vi "Instrument Manager Loop.vi"(8 "System Control":refnum<queue>, 11 "Instrument Manager":refnum<queue>) -> (0 "error out":errorcluster)   [LabVIEW 2020, in "ChromTech Series I Pump.lvlib" / "Instrument Manager.lvlib"]
uses:
  Instrument Manager/Instrument Manager.lvlib
  support/Message Queue/Message Cluster.ctl
  Instrument Manager/Instrument State.ctl
  <vilib>/Utility/error.llb/Error Cluster From Error Code.vi
  <vilib>/ErrorRing/Error Ring.xnode
  support/Message Queue/Message Queue.lvlib
  ChromTech Series I Pump.lvlib
  <instrlib>/RxnRover/ChromtechSeriesIDriver/ChromTech Series I Drivers.lvlib
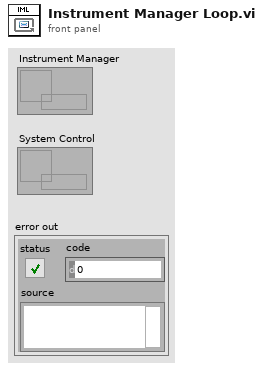
[diagram p1: front panel]
types:
  T1 = typedef "ChromTech Series I Pump.lvlib/Instrument Manager.lvlib/Instrument State.ctl" = cluster{"VISA Resource":refnum<visa-resource-name>, "Flow Rate":dbl, "Running":bool, "Running Since":timestamp, "Pressure Data Point":cluster{"Time Stamp":timestamp, "Value":dbl}, "Upper Pressure Fault":bool, "Lower Pressure Fault":bool, "Motor Stall Fault":bool, "Sampling Rate (sec/sample)":dbl, "Retry Attempts":i32, "Fast Comms":bool}
  T2 = cluster{"seconds since 1Jan1904":timestamp, "Pressure":dbl}
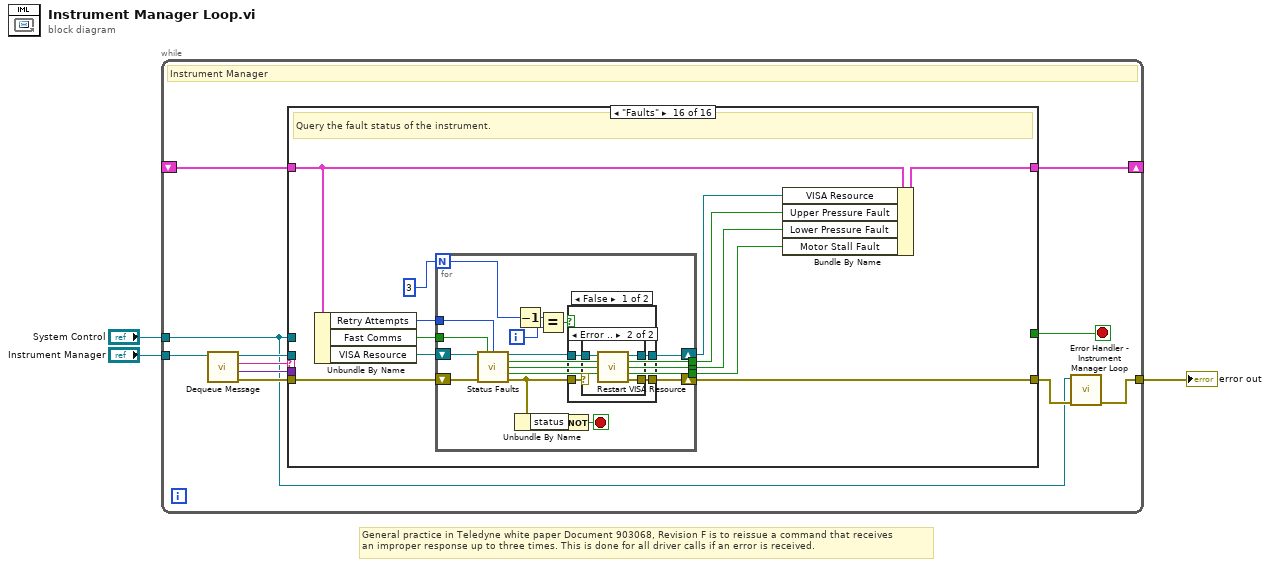
[diagram p0: block diagram]
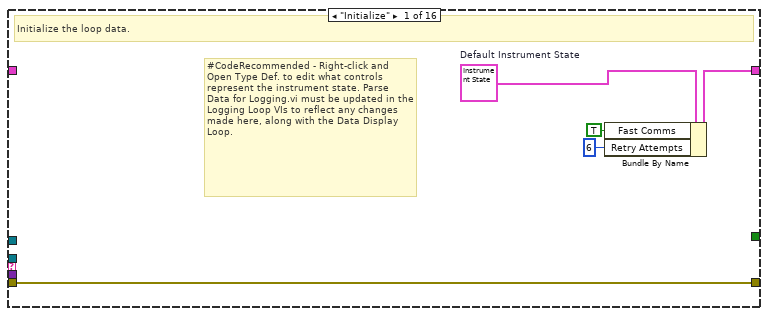
[diagram p2: hidden frame]
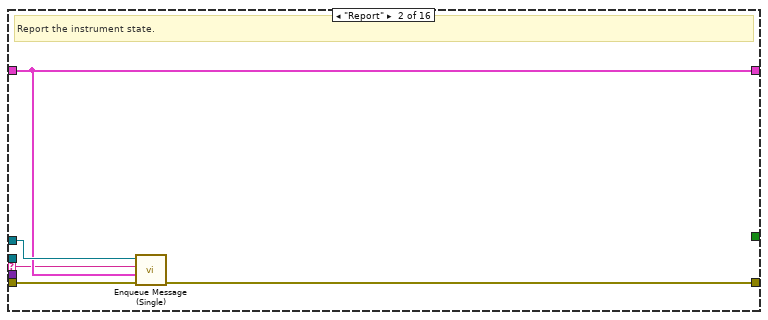
[diagram p3: hidden frame]
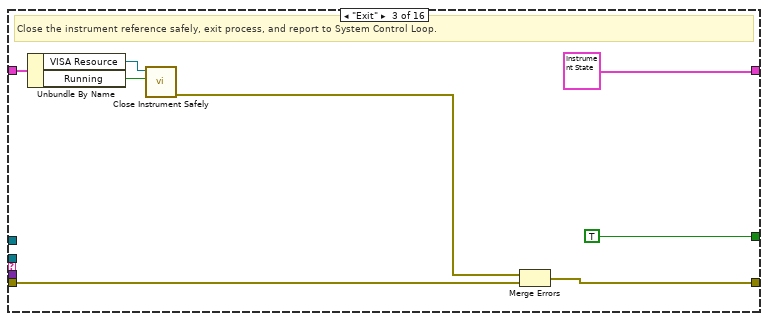
[diagram p4: hidden frame]
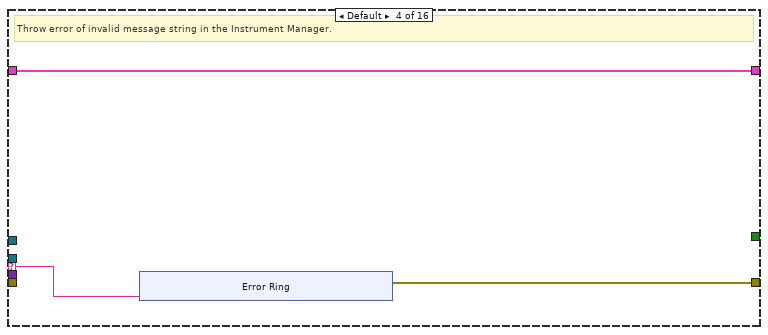
[diagram p5: hidden frame]
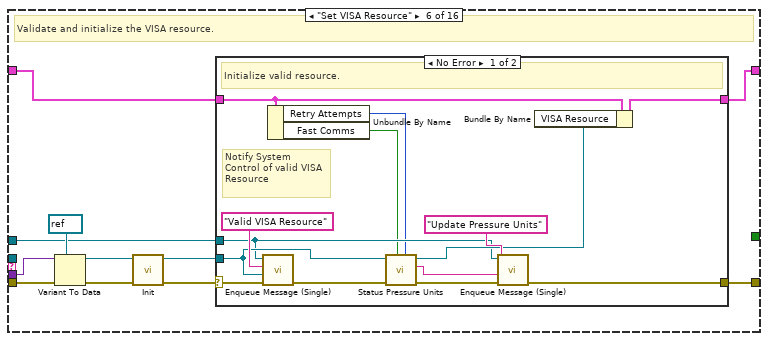
[diagram p7: hidden frame]
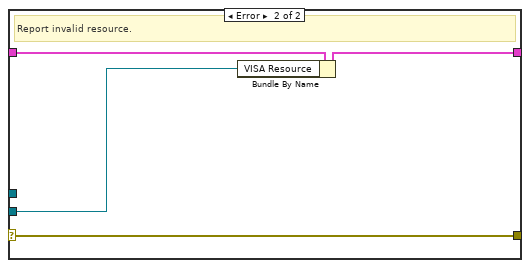
[diagram p8: hidden frame]
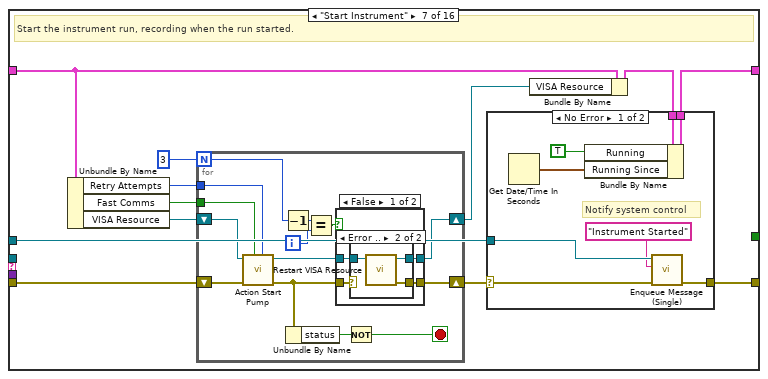
[diagram p9: hidden frame]
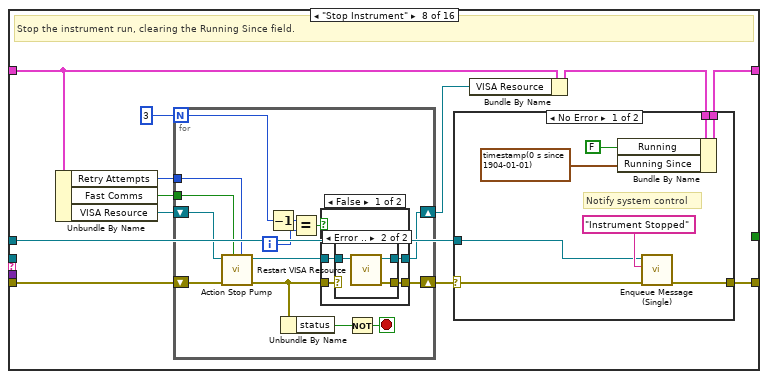
[diagram p13: hidden frame]
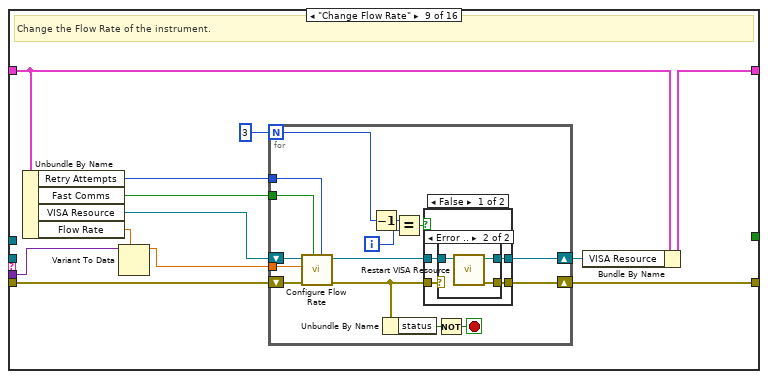
[diagram p17: hidden frame]
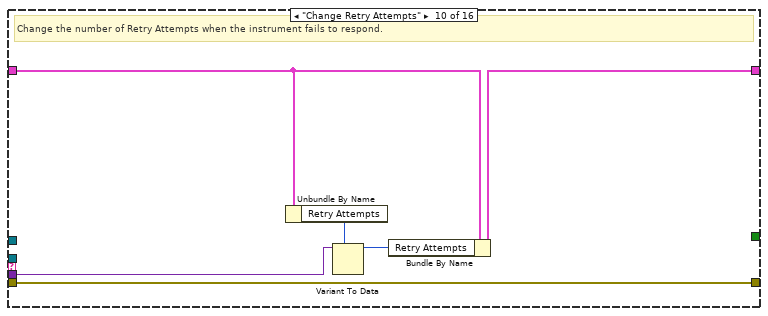
[diagram p20: hidden frame]
diagram:
  # "General practice in Teledyne white paper Document 903068, Revision F is to reissue a command that receives\nan improper response up to three times. This is done for all driver calls if an error is received."
  n1 = while {
    tunnel: "Instrument Manager" -> [w14]
    tunnel: "System Control" -> [w4]
    tunnel: [w8] -> w1
    shift-right: [w6] -> _
    shift-left: _ -> [w7]
    stop <- w5 stop-if-true
    # "Instrument Manager"
    n2 = call "Dequeue Message.vi"("Message Queue"=w14) -> ("error out"=w10:errorcluster, "Message Data"=w11:variant, "Message"=w13:string, "dup Message Queue"=w12:refnum<queue>)  [unwired: 7 in]
    n3 = case shown="\"Faults\"" w13 {
      selector: w13 -> [_ w20 _ w34 _ _ _ _ _ _ _ _ _ _ _ _]
      tunnel: w12 -> [_ _ _ _ _ _ _ _ _ _ _ _ _ _ _ _]
      tunnel: w4 -> [_ w23 _ _ _ w45 w84 w131 _ _ _ _ _ _ _ _]
      tunnel: w11 -> [_ _ _ _ _ w52 _ _ w178 w210 w216 _ _ _ _ _]
      tunnel: w10 -> [w18 w24 w27 _ w43 w51 w82 w129 w173 w207 w213 w220 w229 w264 w304 w342]
      tunnel: [w18 w22 w26 w33 w43 w55 w85 w132 w172 w207 w213 w220 w228 w263 w302 w340] -> w9
      tunnel: w7 -> [_ w21 w32 w35 w44 w54 w81 w127 w177 w209 w215 w219 w227 w265 w301 w339]
      tunnel: [w17 w21 T1 {"VISA Resource"="", "Flow Rate"=0.0, "Running"=FALSE, "Running Since"=timestamp(0 s since 1904-01-01), "Pressure Data Point"={"Time Stamp"=timestamp(0 s since 1904-01-01), "Value"=0.0}, "Upper Pressure Fault"=FALSE, "Lower Pressure Fault"=FALSE, "Motor Stall Fault"=FALSE, "Sampling Rate (sec/sample)"=0.0, "Retry Attempts"=0, "Fast Comms"=FALSE} w35 w44 w53 w83 w130 w179 w211 w217 w219 w230 w268 w303 w341] -> w6
      tunnel: [_ _ TRUE _ _ _ _ _ _ _ _ _ _ _ _ _] -> w5
      frame "Initialize" {
        w19 = T1 {"VISA Resource"="", "Flow Rate"=0.0, "Running"=FALSE, "Running Since"=timestamp(0 s since 1904-01-01), "Pressure Data Point"={"Time Stamp"=timestamp(0 s since 1904-01-01), "Value"=0.0}, "Upper Pressure Fault"=FALSE, "Lower Pressure Fault"=FALSE, "Motor Stall Fault"=FALSE, "Sampling Rate (sec/sample)"=0.0, "Retry Attempts"=0, "Fast Comms"=FALSE}  # Default Instrument State
        # "#CodeRecommended - Right-click and Open Type Def. to edit what controls represent the instrument state. Parse Data for Logging.vi must be updated in the Logging Loop VIs to reflect any changes made here, along with the Data Display Loop."
        # "Initialize the loop data."
        n4 = Bundle By Name(cluster=w19, "Fast Comms"=TRUE, "Retry Attempts"=6) -> (w17:T1)
      }
      frame "Report" {
        # "Report the instrument state."
        n5 = call "Enqueue Message (Single).vi"("error in (no error)"=w24, "Message Data"=w21, "Message"=w20, "Message Queue"=w23) -> ("error out"=w22:errorcluster)  [unwired: 6 in, 1 out]
      }
      frame "Exit" {
        # "Close the instrument reference safely, exit process, and report to System Control Loop."
        n6 = Unbundle By Name(w32) -> ("VISA Resource"=w30:refnum<visa-resource-name>, "Running"=w31:bool)
        n7 = call "Close Instrument Safely.vi"("Running (F)"=w31, "VISA Refnum in"=w30) -> ("error out"=w25:errorcluster)  [unwired: 9 in]
        n8 = Merge Errors(w25, w27) -> (w26:errorcluster)
      }
      frame Default {
        # "Throw error of invalid message string in the Instrument Manager."
        n9 = xnode "Error Ring"("parameter 0"=w34) -> ("error out"=w33:errorcluster)
      }
      frame "--- Copy This Frame ---" {
        # "Copy this frame and add responses to instrument specific messages."
      }
      frame "Set VISA Resource" {
        # "Validate and initialize the VISA resource."
        n10 = Variant To Data(error in=w51, type=refnum<visa-resource-name> refnum, Variant=w52) -> (data=w49:refnum<visa-resource-name>, error out=w50:errorcluster)
        n11 = call "Init.vi"("error in (no error)"=w50, "VISA resource in"=w49) -> ("error out"=w46:errorcluster, "VISA resource out"=w47:refnum<visa-resource-name>)  [unwired: 8 in]
        n12 = case shown="No Error" w46 {
          selector: w46 -> [w69 w70]
          tunnel: w47 -> [w62 w71]
          tunnel: [w64 w70] -> w55
          tunnel: w54 -> [w58 w73]
          tunnel: [w67 w72] -> w53
          tunnel: w45 -> [w60 _]
          frame No Error {
            # "Notify System Control of valid VISA Resource"
            # "Initialize valid resource."
            n13 = call "Enqueue Message (Single).vi"("error in (no error)"=w69, "Message Data"=w62, "Message"="Valid VISA Resource", "Message Queue"=w60) -> ("error out"=w66:errorcluster)  [unwired: 6 in, 1 out]
            n14 = Unbundle By Name(w58) -> ("Retry Attempts"=w57:i32, "Fast Comms"=w56:bool)
            n15 = call <instrlib>:"Status Pressure Units.vi"("Retry Attempts (0)"=w57, "Fast Comms (F)"=w56, "error in (no error)"=w66, "VISA resource name"=w62) -> ("error out"=w65:errorcluster, "Pressure Units"=w59:string, "VISA resource name out"=w61:refnum<visa-resource-name>)  [unwired: 5 in]
            n16 = call "Enqueue Message (Single).vi"("error in (no error)"=w65, "Message Data"=w59, "Message"="Update Pressure Units", "Message Queue"=w60) -> ("error out"=w64:errorcluster)  [unwired: 6 in, 1 out]
            n17 = Bundle By Name(cluster=w58, "VISA Resource"=w61) -> (w67:T1)
          }
          frame Error {
            # "Report invalid resource."
            n18 = Bundle By Name(cluster=w73, "VISA Resource"=w71) -> (w72:T1)
          }
        }
      }
      frame "Start Instrument" {
        # "Start the instrument run, recording when the run started."
        n19 = Unbundle By Name(w81) -> ("Retry Attempts"=w77:i32, "Fast Comms"=w78:bool, "VISA Resource"=w80:refnum<visa-resource-name>)
        n20 = for {
          N: 3 -> [w89]
          tunnel: w78 -> [w97]
          tunnel: w77 -> [w96]
          shift-right: [w86] -> w79
          shift-left: w82 -> [w99]
          shift-right: [w90] -> w74
          shift-left: w80 -> [w98]
          i -> [w88]
          stop <- w94 stop-if-true
          n21 = call <instrlib>:"Action Start Pump.vi"("Retry Attempts (0)"=w96, "Fast Comms (F)"=w97, "error in"=w99, "VISA resource name"=w98) -> ("error out"=w87:errorcluster, "VISA resource name out"=w91:refnum<visa-resource-name>)  [unwired: 6 in]
          n22 = Decrement(x=w89) -> (x-1=w93:i32)
          n23 = Unbundle By Name(w87) -> ("status"=w95:bool)
          n24 = Equal?(x=w93, y=w88) -> (x = y?=w92:bool)
          n25 = case shown="False" w92 {
            tunnel: [w103 w110] -> w86
            tunnel: w91 -> [w102 w109]
            tunnel: w87 -> [w101 w110]
            tunnel: [w100 w109] -> w90
            frame False {
              n26 = case shown="Error .." w101 {
                selector: w101 -> [w105 _]
                tunnel: [w105 w108] -> w103
                tunnel: w102 -> [w104 w107]
                tunnel: [w104 w106] -> w100
                frame No Error {
                }
                frame Error {
                  n27 = call "Restart VISA Resource.vi"("VISA Refnum in"=w107) -> ("error out"=w108:errorcluster, "VISA resource name out"=w106:refnum<visa-resource-name>)  [unwired: 9 in]
                }
              }
            }
            frame True {
            }
          }
          n28 = Not(x=w95) -> (.not. x?=w94:bool)
        }
        n29 = Bundle By Name(cluster=w81, "VISA Resource"=w74) -> (w75:T1)
        n30 = case shown="No Error" w79 {
          selector: w79 -> [w111 w120]
          tunnel: [w118 w120] -> w85
          tunnel: w84 -> [w117 _]
          tunnel: [w115 w119] -> w83
          tunnel: w75 -> [w112 w119]
          frame No Error {
            # "Notify system control"
            n31 = Get Date/Time In Seconds() -> (seconds since 1Jan1904=w113:timestamp)
            n32 = Bundle By Name(cluster=w112, "Running"=TRUE, "Running Since"=w113) -> (w115:T1)
            n33 = call "Enqueue Message (Single).vi"("error in (no error)"=w111, "Message"="Instrument Started", "Message Queue"=w117) -> ("error out"=w118:errorcluster)  [unwired: 7 in, 1 out]
          }
          frame Error {
          }
        }
      }
      frame "Stop Instrument" {
        # "Stop the instrument run, clearing the Running Since field."
        n34 = Unbundle By Name(w127) -> ("Retry Attempts"=w124:i32, "Fast Comms"=w125:bool, "VISA Resource"=w126:refnum<visa-resource-name>)
        n35 = for {
          N: 3 -> [w135]
          tunnel: w125 -> [w144]
          tunnel: w124 -> [w143]
          shift-right: [w136] -> w128
          shift-left: w129 -> [w146]
          shift-right: [w138] -> w121
          shift-left: w126 -> [w145]
          i -> [w134]
          stop <- w141 stop-if-true
          n36 = call <instrlib>:"Action Stop Pump.vi"("Retry Attempts (0)"=w143, "Fast Comms (F)"=w144, "error in"=w146, "VISA resource name"=w145) -> ("error out"=w137:errorcluster, "VISA resource name out"=w139:refnum<visa-resource-name>)  [unwired: 6 in]
          n37 = Decrement(x=w135) -> (x-1=w140:i32)
          n38 = Unbundle By Name(w137) -> ("status"=w142:bool)
          n39 = Equal?(x=w140, y=w134) -> (x = y?=w133:bool)
          n40 = case shown="False" w133 {
            tunnel: [w150 w157] -> w136
            tunnel: w139 -> [w149 w156]
            tunnel: w137 -> [w148 w157]
            tunnel: [w147 w156] -> w138
            frame False {
              n41 = case shown="Error .." w148 {
                selector: w148 -> [w152 _]
                tunnel: [w152 w155] -> w150
                tunnel: w149 -> [w151 w154]
                tunnel: [w151 w153] -> w147
                frame No Error {
                }
                frame Error {
                  n42 = call "Restart VISA Resource.vi"("VISA Refnum in"=w154) -> ("error out"=w155:errorcluster, "VISA resource name out"=w153:refnum<visa-resource-name>)  [unwired: 9 in]
                }
              }
            }
            frame True {
            }
          }
          n43 = Not(x=w142) -> (.not. x?=w141:bool)
        }
        n44 = Bundle By Name(cluster=w127, "VISA Resource"=w121) -> (w122:T1)
        n45 = case shown="No Error" w128 {
          selector: w128 -> [w158 w167]
          tunnel: w122 -> [w165 w166]
          tunnel: [w164 w167] -> w132
          tunnel: w131 -> [w162 _]
          tunnel: [w161 w166] -> w130
          frame No Error {
            # "Notify system control"
            n46 = Bundle By Name(cluster=w165, "Running"=FALSE, "Running Since"=timestamp(0 s since 1904-01-01)) -> (w161:T1)
            n47 = call "Enqueue Message (Single).vi"("error in (no error)"=w158, "Message"="Instrument Stopped", "Message Queue"=w162) -> ("error out"=w164:errorcluster)  [unwired: 7 in, 1 out]
          }
          frame Error {
          }
        }
      }
      frame "Change Flow Rate" {
        # "Change the Flow Rate of the instrument."
        n48 = Unbundle By Name(w177) -> ("Retry Attempts"=w171:i32, "Fast Comms"=w170:bool, "VISA Resource"=w175:refnum<visa-resource-name>, "Flow Rate"=w176:dbl)
        n49 = Variant To Data(type=w176, Variant=w178) -> (data=w174:dbl)  [unwired: 1 in, 1 out]
        n50 = for {
          N: 3 -> [w182]
          tunnel: w174 -> [w193]
          tunnel: w171 -> [w192]
          tunnel: w170 -> [w191]
          shift-right: [w185] -> w172
          shift-left: w173 -> [w190]
          shift-right: [w183] -> w168
          shift-left: w175 -> [w194]
          i -> [w181]
          stop <- w188 stop-if-true
          n51 = call <instrlib>:"Configure Flow Rate.vi"("Retry Attempts (0)"=w192, "Fast Comms (F)"=w191, "error in"=w190, "Flow Input (ml/min)"=w193, "VISA resource name"=w194) -> ("error out"=w186:errorcluster, "VISA resource name out"=w184:refnum<visa-resource-name>)  [unwired: 5 in]
          n52 = Decrement(x=w182) -> (x-1=w187:i32)
          n53 = Unbundle By Name(w186) -> ("status"=w189:bool)
          n54 = Equal?(x=w187, y=w181) -> (x = y?=w180:bool)
          n55 = case shown="False" w180 {
            tunnel: [w198 w205] -> w185
            tunnel: w184 -> [w197 w204]
            tunnel: w186 -> [w196 w205]
            tunnel: [w195 w204] -> w183
            frame False {
              n56 = case shown="Error .." w196 {
                selector: w196 -> [w200 _]
                tunnel: [w200 w203] -> w198
                tunnel: w197 -> [w199 w202]
                tunnel: [w199 w201] -> w195
                frame No Error {
                }
                frame Error {
                  n57 = call "Restart VISA Resource.vi"("VISA Refnum in"=w202) -> ("error out"=w203:errorcluster, "VISA resource name out"=w201:refnum<visa-resource-name>)  [unwired: 9 in]
                }
              }
            }
            frame True {
            }
          }
          n58 = Not(x=w189) -> (.not. x?=w188:bool)
        }
        n59 = Bundle By Name(cluster=w177, "VISA Resource"=w168) -> (w179:T1)
      }
      frame "Change Retry Attempts" {
        # "Change the number of Retry Attempts when the instrument fails to respond."
        n60 = Unbundle By Name(w209) -> ("Retry Attempts"=w206:i32)
        n61 = Variant To Data(type=w206, Variant=w210) -> (data=w208:i32)  [unwired: 1 in, 1 out]
        n62 = Bundle By Name(cluster=w209, "Retry Attempts"=w208) -> (w211:T1)
      }
      frame "Change Fast Comms" {
        # "Change whether to use a return character ('\\r', 0x0D) at the end of each message to the pump. The return character will terminate the write commands to avoid delays by the pump waiting for partial commands."
        n63 = Unbundle By Name(w215) -> ("Fast Comms"=w212:bool)
        n64 = Variant To Data(type=w212, Variant=w216) -> (data=w214:bool)  [unwired: 1 in, 1 out]
        n65 = Bundle By Name(cluster=w215, "Fast Comms"=w214) -> (w217:T1)
      }
      frame "--- Copy for Get State Messages ---" {
        # "Wait 100 ms because if two commands are sent in quick succession, the second will fail."
        # "#CodeNeeded - Use the Bundle by Name function to bundle the new state value into the Instrument State cluster."
        # "#CodeNeeded - Add instrument driver call to query the instrument state requested"
        # "Duplicate this case for messages cases that will query the instrument state."
        n66 = Wait (ms)(milliseconds to wait=u32 100) -> ()  [unwired: 1 out]
      }
      frame "Run State" {
        # "Query the run state of the instrument."
        n67 = Unbundle By Name(w227) -> ("Retry Attempts"=w224:i32, "Fast Comms"=w223:bool, "VISA Resource"=w226:refnum<visa-resource-name>)
        n68 = for {
          N: 3 -> [w232]
          tunnel: [w244] -> w225
          tunnel: w224 -> [w243]
          tunnel: w223 -> [w242]
          shift-right: [w236] -> w228
          shift-left: w229 -> [w241]
          shift-right: [w234] -> w221
          shift-left: w226 -> [w245]
          i -> [w233]
          stop <- w239 stop-if-true
          n69 = call <instrlib>:"Status Run State.vi"("Retry Attempts (0)"=w243, "Fast Comms (F)"=w242, "error in (no error)"=w241, "VISA resource name"=w245) -> ("error out"=w237:errorcluster, "Running?"=w244:bool, "VISA resource name out"=w235:refnum<visa-resource-name>)  [unwired: 5 in]
          n70 = Decrement(x=w232) -> (x-1=w238:i32)
          n71 = Unbundle By Name(w237) -> ("status"=w240:bool)
          n72 = Equal?(x=w238, y=w233) -> (x = y?=w231:bool)
          n73 = case shown="False" w231 {
            tunnel: [w249 w256] -> w236
            tunnel: w235 -> [w248 w255]
            tunnel: w237 -> [w247 w256]
            tunnel: [w246 w255] -> w234
            frame False {
              n74 = case shown="Error .." w247 {
                selector: w247 -> [w251 _]
                tunnel: [w251 w254] -> w249
                tunnel: w248 -> [w250 w253]
                tunnel: [w250 w252] -> w246
                frame No Error {
                }
                frame Error {
                  n75 = call "Restart VISA Resource.vi"("VISA Refnum in"=w253) -> ("error out"=w254:errorcluster, "VISA resource name out"=w252:refnum<visa-resource-name>)  [unwired: 9 in]
                }
              }
            }
            frame True {
            }
          }
          n76 = Not(x=w240) -> (.not. x?=w239:bool)
        }
        n77 = Bundle By Name(cluster=w227, "VISA Resource"=w221, "Running"=w225) -> (w230:T1)
      }
      frame "Pressure" {
        # "Query the pressure value of the instrument."
        n78 = Unbundle By Name(w265) -> ("Retry Attempts"=w259:i32, "Fast Comms"=w260:bool, "VISA Resource"=w262:refnum<visa-resource-name>)
        n79 = for {
          N: 3 -> [w270]
          tunnel: [w282] -> w261
          tunnel: w260 -> [w281]
          tunnel: w259 -> [w280]
          shift-right: [w274] -> w263
          shift-left: w264 -> [w279]
          shift-right: [w272] -> w257
          shift-left: w262 -> [w283]
          i -> [w271]
          stop <- w277 stop-if-true
          n80 = call <instrlib>:"Status Get Pressure.vi"("Retry Attempts (0)"=w280, "Fast Comms (F)"=w281, "error in"=w279, "VISA resource name"=w283) -> ("error out"=w275:errorcluster, "Pressure"=w282:dbl, "VISA resource name out"=w273:refnum<visa-resource-name>)  [unwired: 5 in]
          n81 = Decrement(x=w270) -> (x-1=w276:i32)
          n82 = Unbundle By Name(w275) -> ("status"=w278:bool)
          n83 = Equal?(x=w276, y=w271) -> (x = y?=w269:bool)
          n84 = case shown="False" w269 {
            tunnel: [w287 w294] -> w274
            tunnel: w273 -> [w286 w293]
            tunnel: w275 -> [w285 w294]
            tunnel: [w284 w293] -> w272
            frame False {
              n85 = case shown="Error .." w285 {
                selector: w285 -> [w289 _]
                tunnel: [w289 w292] -> w287
                tunnel: w286 -> [w288 w291]
                tunnel: [w288 w290] -> w284
                frame No Error {
                }
                frame Error {
                  n86 = call "Restart VISA Resource.vi"("VISA Refnum in"=w291) -> ("error out"=w292:errorcluster, "VISA resource name out"=w290:refnum<visa-resource-name>)  [unwired: 9 in]
                }
              }
            }
            frame True {
            }
          }
          n87 = Not(x=w278) -> (.not. x?=w277:bool)
        }
        n88 = Get Date/Time In Seconds() -> (seconds since 1Jan1904=w267:timestamp)
        n89 = Bundle("seconds since 1Jan1904"=w267, "Pressure"=w261) -> (w266:T2)  [unwired: 1 in]
        n90 = Bundle By Name(cluster=w265, "Pressure Data Point"=w266, "VISA Resource"=w257) -> (w268:T1)
      }
      frame "Flow Rate" {
        # "Query the flow rate of the instrument."
        n91 = Unbundle By Name(w301) -> ("Retry Attempts"=w298:i32, "Fast Comms"=w297:bool, "VISA Resource"=w300:refnum<visa-resource-name>)
        n92 = for {
          N: 3 -> [w308]
          tunnel: [w318] -> w299
          tunnel: w298 -> [w317]
          tunnel: w297 -> [w316]
          shift-right: [w310] -> w302
          shift-left: w304 -> [w315]
          shift-right: [w305] -> w295
          shift-left: w300 -> [w319]
          i -> [w307]
          stop <- w313 stop-if-true
          n93 = call <instrlib>:"Status Get Flow Rate.vi"("Retry Attempts (0)"=w317, "Fast Comms (F)"=w316, "error in"=w315, "VISA resource name"=w319) -> ("error out"=w311:errorcluster, "Flow Rate"=w318:dbl, "VISA resource name out"=w306:refnum<visa-resource-name>)  [unwired: 5 in]
          n94 = Unbundle By Name(w311) -> ("status"=w314:bool)
          n95 = Decrement(x=w308) -> (x-1=w312:i32)
          n96 = Equal?(x=w312, y=w307) -> (x = y?=w309:bool)
          n97 = case shown="False" w309 {
            tunnel: [w323 w330] -> w310
            tunnel: w306 -> [w322 w329]
            tunnel: w311 -> [w321 w330]
            tunnel: [w320 w329] -> w305
            frame False {
              n98 = case shown="Error .." w321 {
                selector: w321 -> [w325 _]
                tunnel: [w325 w328] -> w323
                tunnel: w322 -> [w324 w327]
                tunnel: [w324 w326] -> w320
                frame No Error {
                }
                frame Error {
                  n99 = call "Restart VISA Resource.vi"("VISA Refnum in"=w327) -> ("error out"=w328:errorcluster, "VISA resource name out"=w326:refnum<visa-resource-name>)  [unwired: 9 in]
                }
              }
            }
            frame True {
            }
          }
          n100 = Not(x=w314) -> (.not. x?=w313:bool)
        }
        n101 = Bundle By Name(cluster=w301, "VISA Resource"=w295, "Flow Rate"=w299) -> (w303:T1)
      }
      frame "Faults" {
        # "Query the fault status of the instrument."
        n102 = Unbundle By Name(w339) -> ("Retry Attempts"=w334:i32, "Fast Comms"=w333:bool, "VISA Resource"=w338:refnum<visa-resource-name>)
        n103 = for {
          N: 3 -> [w345]
          tunnel: [w357] -> w337
          tunnel: [w356] -> w336
          tunnel: [w355] -> w335
          tunnel: w334 -> [w354]
          tunnel: w333 -> [w353]
          shift-right: [w348] -> w340
          shift-left: w342 -> [w359]
          shift-right: [w346] -> w331
          shift-left: w338 -> [w358]
          i -> [w344]
          stop <- w351 stop-if-true
          n104 = call <instrlib>:"Status Faults.vi"("VISA resource name"=w358, "Fast Comms (F)"=w353, "Retry Attempts (0)"=w354, "error in (no error)"=w359) -> ("VISA resource name out"=w347:refnum<visa-resource-name>, "Upper Pressure Fault"=w356:bool, "Lower Pressure Fault"=w357:bool, "Motor Stall Fault"=w355:bool, "error out"=w349:errorcluster)  [unwired: 7 in]
          n105 = Decrement(x=w345) -> (x-1=w350:i32)
          n106 = Unbundle By Name(w349) -> ("status"=w352:bool)
          n107 = Equal?(x=w350, y=w344) -> (x = y?=w343:bool)
          n108 = Not(x=w352) -> (.not. x?=w351:bool)
          n109 = case shown="False" w343 {
            tunnel: [w363 w370] -> w348
            tunnel: w347 -> [w362 w369]
            tunnel: w349 -> [w361 w370]
            tunnel: [w360 w369] -> w346
            frame False {
              n110 = case shown="Error .." w361 {
                selector: w361 -> [w365 _]
                tunnel: [w365 w368] -> w363
                tunnel: w362 -> [w364 w367]
                tunnel: [w364 w366] -> w360
                frame No Error {
                }
                frame Error {
                  n111 = call "Restart VISA Resource.vi"("VISA Refnum in"=w367) -> ("error out"=w368:errorcluster, "VISA resource name out"=w366:refnum<visa-resource-name>)  [unwired: 9 in]
                }
              }
            }
            frame True {
            }
          }
        }
        n112 = Bundle By Name(cluster=w339, "VISA Resource"=w331, "Upper Pressure Fault"=w336, "Lower Pressure Fault"=w337, "Motor Stall Fault"=w335) -> (w341:T1)
      }
    }
    n113 = call "Error Handler - Instrument Manager Loop.vi"("error in (no error)"=w9, "Message Queue"=w4) -> ("dup error in"=w8:errorcluster)  [unwired: 8 in, 1 out]
  }
  "error out" <- w1
